vi "Write Sequence Msg.vi"(10 "Sequence.lvlib:Sequence Msg.lvclass":refnum<class "Sequence Msg.lvclass">, 11 "Sequence in":refnum<class "Sequence.lvclass">) -> (3 "Sequence out":refnum<class "Sequence.lvclass">)   [LabVIEW 2019, in "Sequence.lvlib" / "Sequence.lvclass"]
uses:
  Sequence.lvclass
  Sequence Messages/Sequence Msg/Sequence Msg.lvclass
  Sequence.lvclass/Sequence.ctl
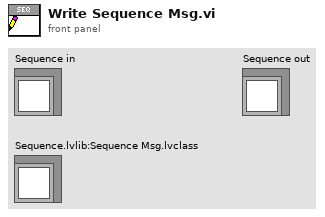
[diagram p1: front panel]
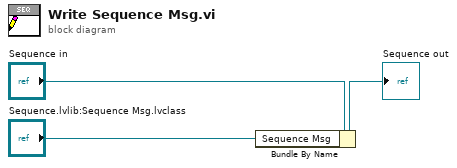
[diagram p0: block diagram]
diagram:
  n1 = Bundle By Name(cluster="Sequence in", "Sequence Msg"="Sequence.lvlib:Sequence Msg.lvclass") -> (→"Sequence out":refnum<class "Sequence.lvclass">)
